vi "SetUp.vi"(8 "error in (no error)":errorcluster, 11 "Prueba08 in":refnum<class "Prueba09.lvclass">) -> (0 "error out":errorcluster, 3 "Prueba08 out":refnum<class "Prueba09.lvclass">)   [LabVIEW 2019, in "Prueba09.lvclass"]
uses:
  Prueba09.lvclass
  Prueba09.lvclass/Prueba09.ctl
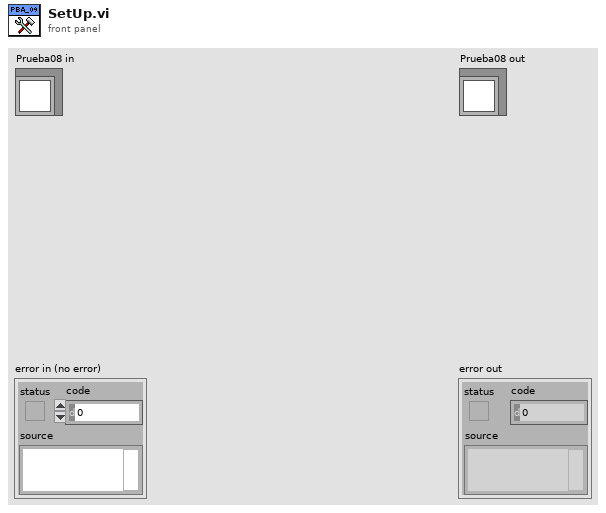
[diagram p1: front panel]
types:
  T1 = typedef "Prueba09.lvclass/BD.ctl" = cluster{"MaxNivelCpeak":dbl, "Incertidumbre":string[], "Tol +":string[], "Tol -":string[]}
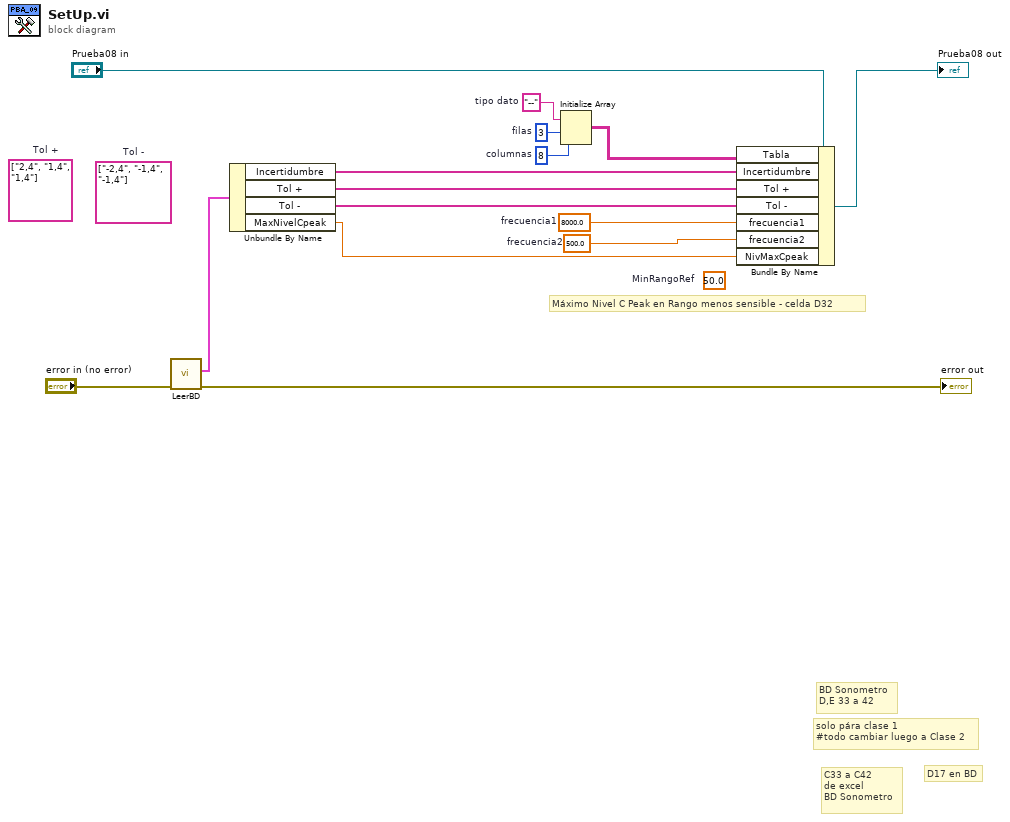
[diagram p0: block diagram]
diagram:
  w7 = 500.0  # frecuencia2
  (unwired) 50.0  # MinRangoRef
  w14 = 8000.0  # frecuencia1
  (unwired) string[] ["-2,4", "-1,4", "-1,4"]  # Tol -
  (unwired) string[] ["2,4", "1,4", "1,4"]  # Tol +
  w12 = 8  # columnas
  w8 = 3  # filas
  w13 = "--"  # tipo dato
  # "Máximo Nivel C Peak en Rango menos sensible - celda D32"
  # "D17 en BD"
  # "BD Sonometro\nD,E 33 a 42"
  # "solo pára clase 1\n#todo cambiar luego a Clase 2"
  # "C33 a C42\nde excel\nBD Sonometro"
  n1 = call "LeerBD.vi"("error in (no error)"="error in (no error)") -> ("error out"=→"error out":errorcluster, "BD"=w5:T1)  [unwired: 8 in, 1 out]
  n2 = Unbundle By Name(w5) -> ("Incertidumbre"=w4:string[], "Tol +"=w3:string[], "Tol -"=w2:string[], "MaxNivelCpeak"=w1:dbl)
  n3 = Initialize Array(w13, w8, w12) -> (w11:string[][])
  n4 = Bundle By Name(cluster="Prueba08 in", "Tabla"=w11, "Incertidumbre"=w4, "Tol +"=w3, "Tol -"=w2, "frecuencia1"=w14, "frecuencia2"=w7, "NivMaxCpeak"=w1) -> (→"Prueba08 out":refnum<class "Prueba09.lvclass">)
